vi "Background_MC_Acquire.vi"(8 "error in":errorcluster, 9 "Image In":T2, 10 "Frames":i16, 11 "FPGA VI Reference In":T1) -> (0 "error out":errorcluster, 2 "Image":T2(plugin-control), 3 "FPGA VI Reference Out":T1)   [LabVIEW 2020]
uses:
  RIG-SPECIFIC FILES/FPGA Refs/FPGA Ref.ctl
  <vilib>/vision/Image Controls.llb/IMAQ Image.ctl
  <vilib>/Utility/error.llb/Error Cluster From Error Code.vi
  <vilib>/rvi/errors/niLvFpgaAdjustHostInterfaceError.vi
  <vilib>/rvi/interface/nirviMethod/nirviMethod.xnode
  <vilib>/FPGAPlugInAG/Dynamic/niLvFpga_ReadFifo_Dynamic.vi
  <vilib>/rvi/errors/niLvFpgaMergeErrorWithErrorCode.vi
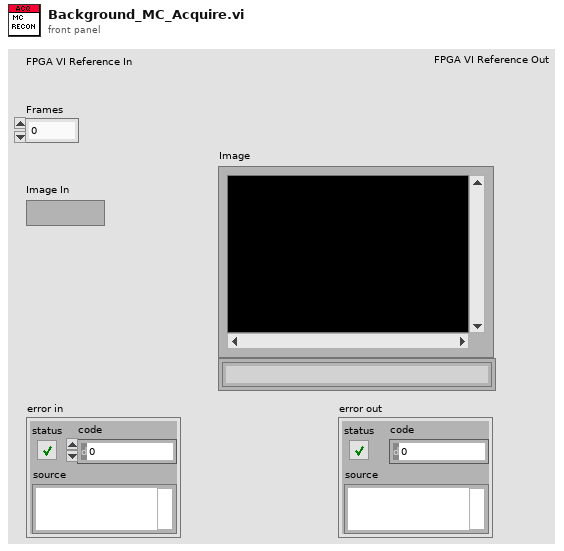
[diagram p1: front panel]
types:
  T1 = typedef "FPGA Ref.ctl" = refnum<k20>
  T2 = typedef "IMAQ Image.ctl" = refnum<image>
  T3 = typedef "Ref DAQ Param.ctl" = cluster{"Full Frame Size":u16, "Ref Field of View":sgl, "Ref Zoom":i8, "Ref_dwellTime":sgl, "Ref X-pixels-per-line(Npxr)":i16, "Ref Y-lines-per-image(Npyr)":i16, "Ref Z-lines-per-image":i16, "Ignore Z lines":i16, "Ref Scan Cycles":i32, "Ref threshold XY":u16, "Ref threshold Z":u16, "Ref average XY":u16, "Ref Average  Z":u16, "Proportional_scale":fxp<+,16,2>, "Integral_scale":fxp<+/-,16,12>, "Proportional_scale Z":fxp<+,16,2>, "Integral_scale Z":fxp<+/-,16,12>, "Diff_threshold":fxp<+,16,2>, "Diff_threshold _z":fxp<+,16,2>, "Sliding Average":bool, "Ref count reset enabled":bool}
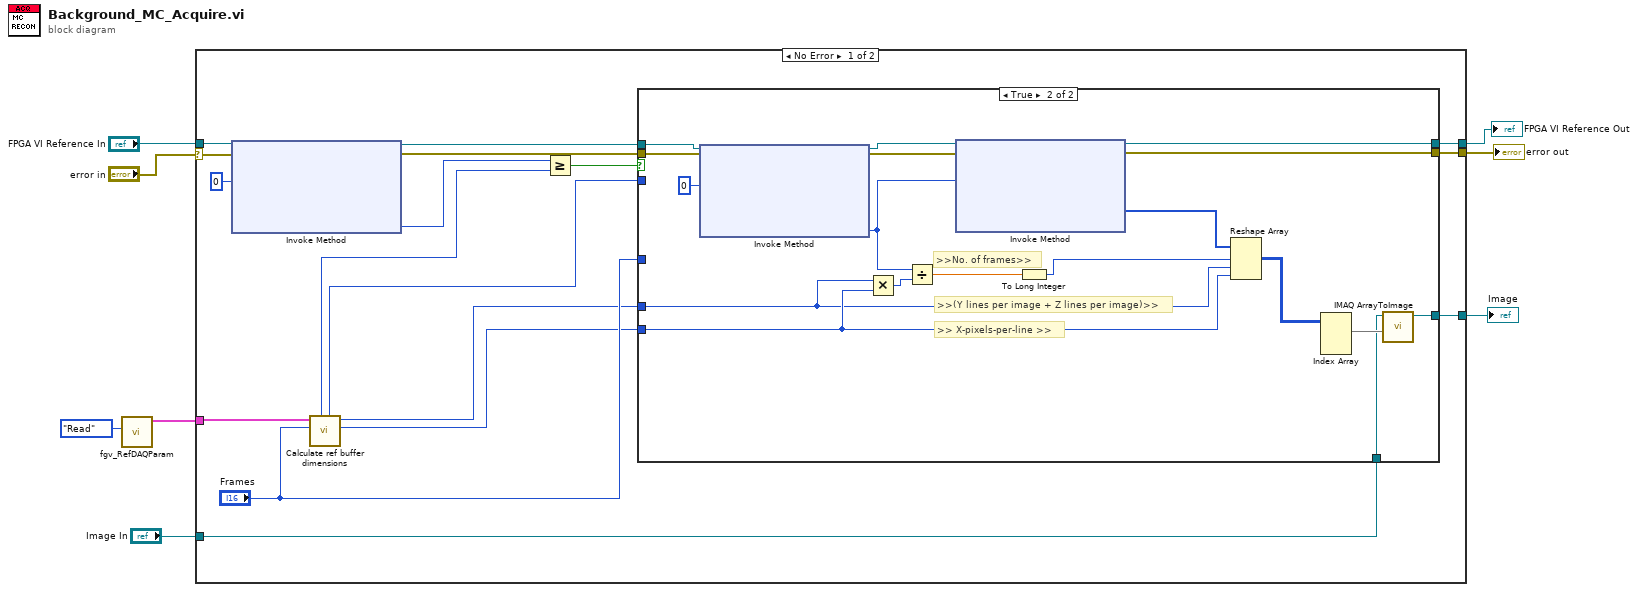
[diagram p0: block diagram]
diagram:
  n1 = call "fgv_RefDAQParam.vi"("Function"=enum16{"Initialize", "Write", "Read"}."Read") -> ("RefDAQParam"=w5:T3)  [unwired: 9 in, 1 out]
  n2 = case shown="No Error" "error in" {
    selector: "error in" -> [w23 w46]
    tunnel: "FPGA VI Reference In" -> [w25 w47]
    tunnel: w5 -> [w18 _]
    tunnel: "Image In" -> [w12 w48]
    tunnel: [w11 w48] -> w3
    tunnel: [w10 w47] -> w2
    tunnel: [w9 w46] -> w1
    frame No Error {
      n3 = xnode "Invoke Method"("FPGA VI Reference In"=w25, "error in"=w23, "Number of Elements"=u32 0) -> ("FPGA VI Reference Out"=w20:T1, "error out"=w19:errorcluster, "Elements Remaining"=w22:u32)  [unwired: 1 in, 1 out]
      n4 = call "Calculate ref buffer dimensions.vi"("Frames"="Frames", "RefDAQParam in"=w18) -> ("Ref X-pixels-per-line(Npxr)"=w13:i16, "Y lines  + Z lines"=w14:i16, "Number of pixels per frame"=w15:i16, "Total number of pixels"=w16:i16)  [unwired: 4 in, 2 out]
      n5 = Greater Or Equal?(x=w22, y=w16) -> (x >= y?=w21:bool)
      n6 = case shown="True" w21 {
        tunnel: w20 -> [w28 w36]
        tunnel: w19 -> [w27 w45]
        tunnel: w15 -> [_ _]
        tunnel: "Frames" -> [_ _]
        tunnel: w14 -> [_ w33]
        tunnel: w13 -> [_ w34]
        tunnel: w12 -> [w26 w41]
        tunnel: [w26 w40] -> w11
        tunnel: [w28 w39] -> w10
        tunnel: [w27 w38] -> w9
        frame False {
        }
        frame True {
          # ">>No. of frames>>"
          # ">>(Y lines per image + Z lines per image)>>"
          # ">> X-pixels-per-line >>"
          n7 = xnode "Invoke Method"("FPGA VI Reference In"=w36, "Number of Elements"=u32 0) -> ("FPGA VI Reference Out"=w37:T1, "Elements Remaining"=w29:u32)  [unwired: 2 in, 2 out]
          n8 = Multiply(x=w33, y=w34) -> (x*y=w32:i16)
          n9 = Divide(x=w29, y=w32) -> (x/y=w30:dbl)
          n10 = xnode "Invoke Method"("FPGA VI Reference In"=w37, "error in"=w45, "Number of Elements"=w29) -> ("FPGA VI Reference Out"=w39:T1, "error out"=w38:errorcluster, "Data"=w44:u16[])  [unwired: 1 in, 1 out]
          n11 = To Long Integer(number=w30) -> (32bit integer=w31:i32)
          n12 = Reshape Array(w44, w31, w33, w34) -> (w42:u16[][][])
          n13 = Index Array(array=w42) -> (element=w43:u16[][])  [unwired: 3 in]
          n14 = call "IMAQ ArrayToImage"("Image Pixels (I16)"=w43, "Image"=w41) -> ("Image Out"=w40:T2)  [unwired: 8 in, 1 out]
        }
      }
    }
    frame Error {
    }
  }
  "Image" <- w3
  "FPGA VI Reference Out" <- w2
  "error out" <- w1
